vi "Get Pin Map ID.vi"(8 "error in":errorcluster, 11 "Sequence Context":refnum<k7>) -> (0 "error out":errorcluster, 3 "pin_map_id":string)   [LabVIEW 2020, in "NIDigitalSPI.lvlib"]
uses:
  NIDigitalSPI.lvlib
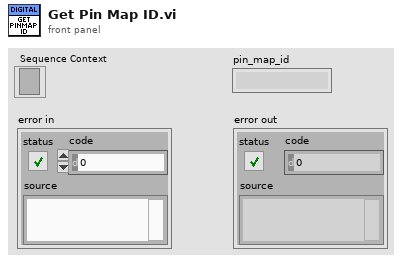
[diagram p1: front panel]
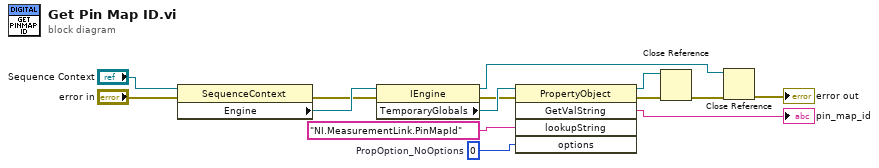
[diagram p0: block diagram]
diagram:
  w5 = 0  # PropOption_NoOptions
  n1 = property class="SequenceContext"(reference="Sequence Context", error in="error in") -> (error out=w7:errorcluster, "Engine"=w8:refnum<k7>)  [unwired: 1 out]
  n2 = property class="IEngine"(reference=w8, error in=w7) -> (reference out=w13:refnum<k7>, error out=w6:errorcluster, "TemporaryGlobals"=w9:refnum<k7>)
  n3 = invoke class="PropertyObject" method="GetValString"(reference=w9, error in=w6, "lookupString"="NI.MeasurementLink.PinMapId", "options"=w5) -> (reference out=w11:refnum<k7>, error out=w12:errorcluster, "GetValString"=→"pin_map_id":string)  [unwired: 1 in, 2 out]
  n4 = Close Reference(reference=w11, error in (no error)=w12) -> (error out=w14:errorcluster)
  n5 = Close Reference(reference=w13, error in (no error)=w14) -> (error out=→"error out":errorcluster)
